vi "CH0_write_byte_data_and_sign_into_mem_no_g_Rev02x.vi"(0 "MB data":u8, 1 "UB data":u8, 2 "Address of the sign":string, 3 "USB Interface Name":refnum<visa-resource-name>="COM3", 4 "HB data":u8, 5 "LB data":u8, 6 "MB address":string, 7 "HB address":string, 8 "Sign Value":dbl, 9 "WRITE DATA":bool, 10 "Input buffer size":u32=16384, 11 "LB address":string, 12 "UB address":string, 13 "error in (no error)":errorcluster) -> (14 "MB data string":string, 15 "UB data string":string, 17 "error out":errorcluster, 18 "HB data string":string, 19 "LB data string":string)   [LabVIEW 2012]
panel:
  out "T command Bytes sent 5":dbl
  out "T command Bytes sent 4":dbl
  out "T command Bytes sent 3":dbl
  out "T command Bytes sent 2":dbl
  out "T command Bytes sent":dbl
  out "First 'T' Number of bytes written":dbl
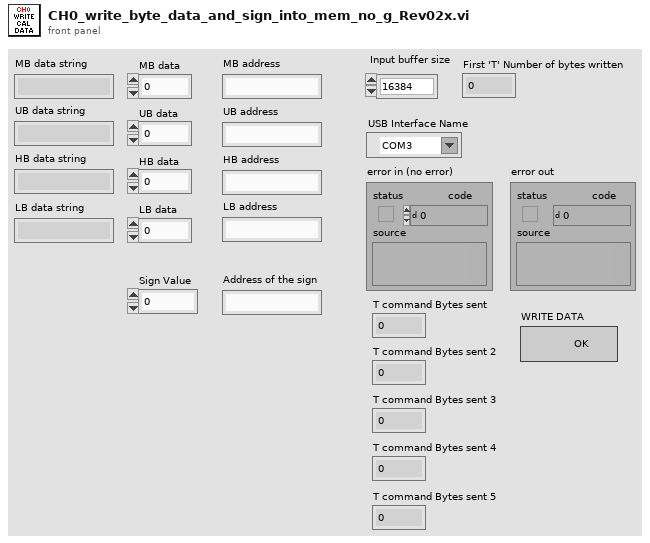
[diagram p1: front panel]
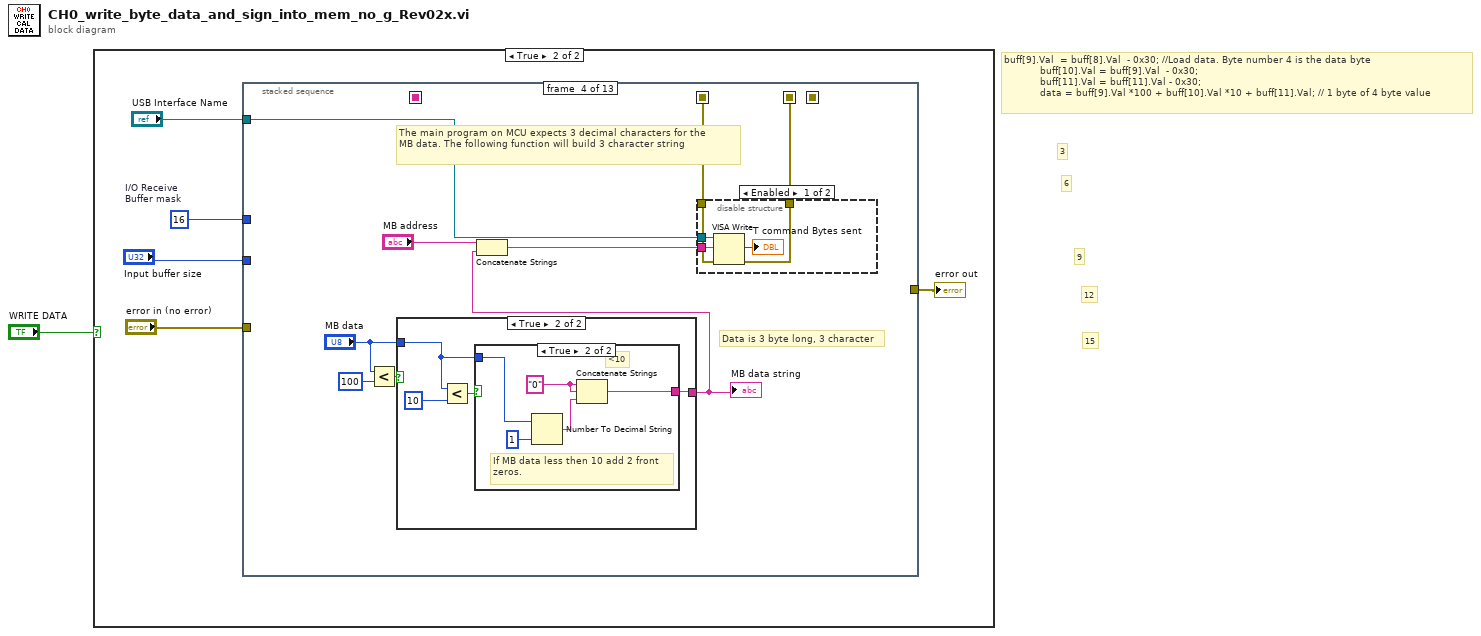
[diagram p0: block diagram]
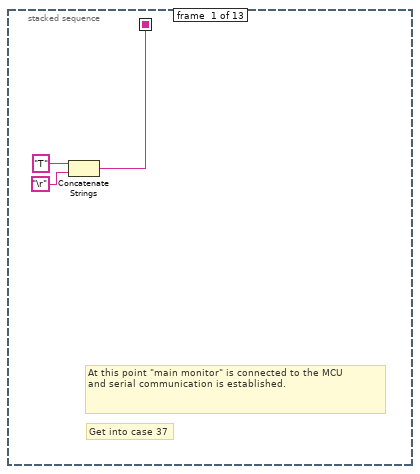
[diagram p3: hidden frame]
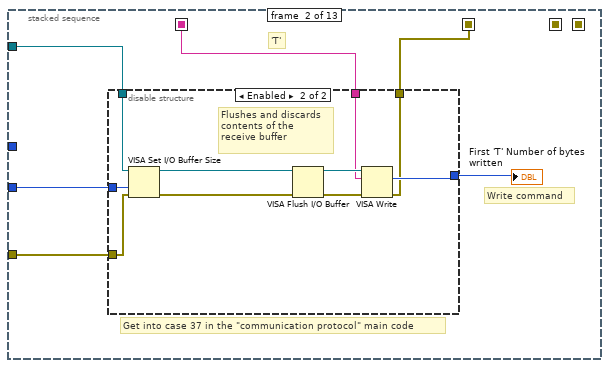
[diagram p4: hidden frame]
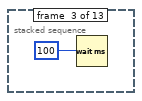
[diagram p6: hidden frame]
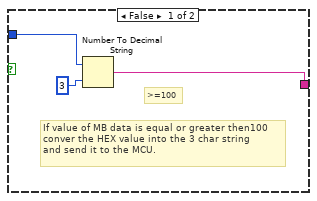
[diagram p7: hidden frame]
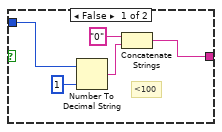
[diagram p8: hidden frame]
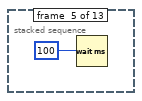
[diagram p10: hidden frame]
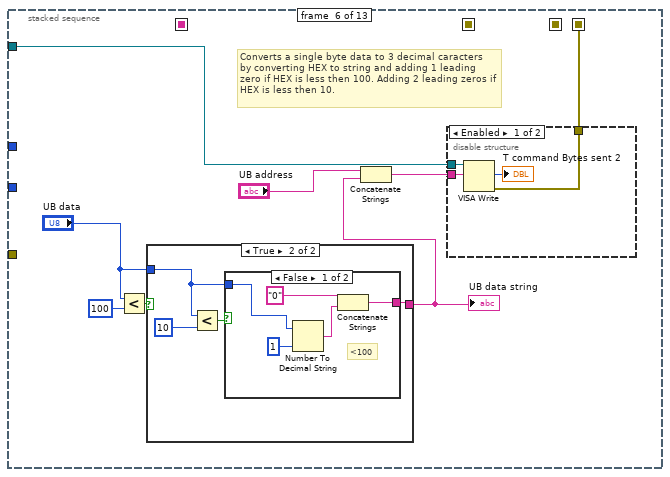
[diagram p11: hidden frame]
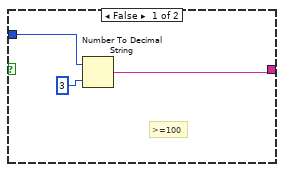
[diagram p12: hidden frame]
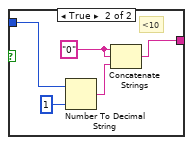
[diagram p13: hidden frame]
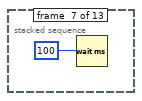
[diagram p15: hidden frame]
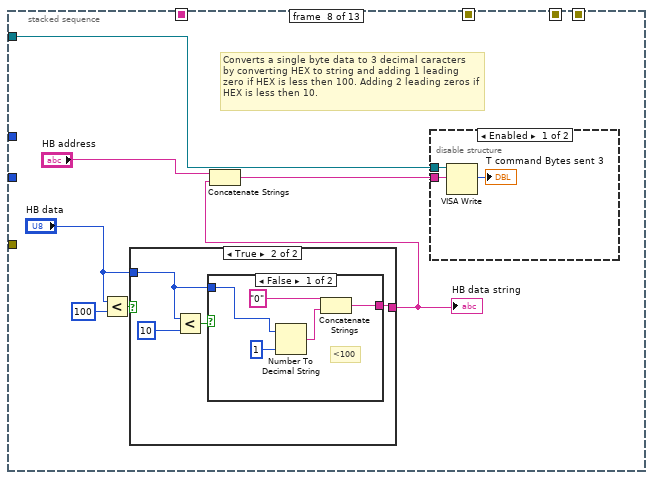
[diagram p16: hidden frame]
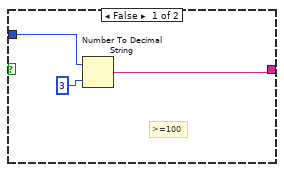
[diagram p17: hidden frame]
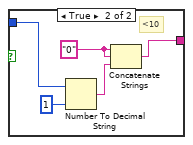
[diagram p18: hidden frame]
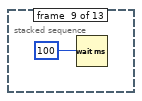
[diagram p20: hidden frame]
diagram:
  # "15"
  # "3"
  # "12"
  # "9"
  # "6"
  # "buff[9].Val  = buff[8].Val  - 0x30; //Load data. Byte number 4 is the data byte           \n            buff[10].Val = buff[9].Val  - 0x30;           \n            buff[11].Val = buff[11].Val - 0x30;               \n            data = buff[9].Val *100 + buff[10].Val *10 + buff[11].Val; // 1 byte of 4 byte value"
  n1 = case shown="True" "WRITE DATA" {
    frame False {
    }
    frame True {
      w4 = u16 16  # I/O Receive Buffer mask
      n2 = stacked-sequence {
        seq-local: [w7 _ _ _ _ _ _ _ _ _ _ _ _] -> [_ w12 _ _ _ _ _ _ _ _ _ _ _]
        seq-local: [_ w11 _ _ _ _ _ _ _ _ _ _ _] -> [_ _ _ w29 _ _ _ _ _ _ _ _ _]
        seq-local: [_ _ _ w28 _ _ _ _ _ _ _ _ _] -> [_ _ _ _ _ _ _ _ _ _ _ _ _]
        seq-local: [_ _ _ _ _ w60 _ _ _ _ _ _ _] -> [_ _ _ _ _ _ _ _ _ _ _ _ _]
        tunnel: "USB Interface Name" -> [_ w15 _ w34 _ w61 _ w90 _ w119 _ w153 w159]
        tunnel: "error in (no error)" -> [_ w14 _ _ _ _ _ _ _ _ _ _ _]
        tunnel: "Input buffer size" -> [_ w13 _ _ _ _ _ _ _ _ _ _ _]
        tunnel: w4 -> [_ _ _ _ _ _ _ _ _ _ _ _ _]
        tunnel: [_ _ _ _ _ _ _ _ _ w117 _ _ _] -> w3
        frame #0 {
          # "At this point \"main monitor\" is connected to the MCU\nand serial communication is established."
          # "Get into case 37"
          n3 = Concatenate Strings("T", "\r") -> (w7:string)
        }
        frame #1 {
          # "'T'"
          # "Get into case 37 in the \"communication protocol\" main code"
          # "Write command"
          n4 = disable-structure shown="Enabled" {
            disable-tunnel: w13 -> [_ w21]
            disable-tunnel: w12 -> [_ w20]
            disable-tunnel: w15 -> [_ w19]
            disable-tunnel: w14 -> [_ w18]
            disable-tunnel: [_ w17] -> w10
            disable-tunnel: [_ w16] -> w11
            frame Disabled {
            }
            frame Enabled {
              # "Flushes and discards \ncontents of the \nreceive buffer"
              n5 = VISA Set I/O Buffer Size(VISA resource name=w19, size (4096)=w21, error in (no error)=w18) -> (VISA resource name out=w23:refnum<visa-resource-name>, error out=w22:errorcluster)  [unwired: 1 in]
              n6 = VISA Flush I/O Buffer(VISA resource name=w23, error in (no error)=w22) -> (VISA resource name out=w25:refnum<visa-resource-name>, error out=w24:errorcluster)  [unwired: 1 in]
              n7 = VISA Write(VISA resource name=w25, write buffer=w20, error in (no error)=w24) -> (return count=w17:u32, error out=w16:errorcluster)  [unwired: 1 out]
            }
          }
          "First 'T' Number of bytes written" <- w10
        }
        frame #2 {
          n8 = Wait (ms)(milliseconds to wait=100) -> ()  [unwired: 1 out]
        }
        frame #3 {
          # "Data is 3 byte long, 3 character"
          # "The main program on MCU expects 3 decimal characters for the \nMB data. The following function will build 3 character string"
          n9 = Less?(x="MB data", y=100) -> (x < y?=w33:bool)
          n10 = case shown="True" w33 {
            tunnel: [w38 w39] -> w30
            tunnel: "MB data" -> [w36 w40]
            frame False {
              # "If value of MB data is equal or greater then100\nconver the HEX value into the 3 char string \nand send it to the MCU."
              # ">=100"
              n11 = Number To Decimal String(number=w36, width (-)=3) -> (decimal integer string=w38:string)
            }
            frame True {
              n12 = Less?(x=w40, y=10) -> (x < y?=w42:bool)
              n13 = case shown="True" w42 {
                tunnel: w40 -> [w45 w48]
                tunnel: [w44 w49] -> w39
                frame False {
                  # "<100"
                  n14 = Number To Decimal String(number=w45, width (-)=1) -> (decimal integer string=w46:string)
                  n15 = Concatenate Strings("0", w46) -> (w44:string)
                }
                frame True {
                  w50 = "0"
                  # "If MB data less then 10 add 2 front\nzeros."
                  # "<10"
                  n16 = Number To Decimal String(number=w48, width (-)=1) -> (decimal integer string=w51:string)
                  n17 = Concatenate Strings(w50, w50, w51) -> (w49:string)
                }
              }
            }
          }
          "MB data string" <- w30
          n18 = Concatenate Strings("MB address", w30) -> (w35:string)
          n19 = disable-structure shown="Enabled" {
            disable-tunnel: w35 -> [w56 _]
            disable-tunnel: w34 -> [w55 _]
            disable-tunnel: w29 -> [w54 _]
            disable-tunnel: [w53 _] -> w28
            frame Enabled {
              n20 = VISA Write(VISA resource name=w55, write buffer=w56, error in (no error)=w54) -> (return count=→"T command Bytes sent":u32, error out=w53:errorcluster)  [unwired: 1 out]
            }
            frame Disabled {
            }
          }
        }
        frame #4 {
          n21 = Wait (ms)(milliseconds to wait=100) -> ()  [unwired: 1 out]
        }
        frame #5 {
          # "Converts a single byte data to 3 decimal caracters\nby converting HEX to string and adding 1 leading zero if HEX is less then 100. Adding 2 leading zeros if HEX is less then 10."
          n22 = Less?(x="UB data", y=100) -> (x < y?=w65:bool)
          n23 = case shown="True" w65 {
            tunnel: [w69 w70] -> w62
            tunnel: "UB data" -> [w67 w71]
            frame False {
              # ">=100"
              n24 = Number To Decimal String(number=w67, width (-)=3) -> (decimal integer string=w69:string)
            }
            frame True {
              n25 = Less?(x=w71, y=10) -> (x < y?=w73:bool)
              n26 = case shown="False" w73 {
                tunnel: w71 -> [w75 w79]
                tunnel: [w74 w80] -> w70
                frame False {
                  # "<100"
                  n27 = Number To Decimal String(number=w75, width (-)=1) -> (decimal integer string=w76:string)
                  n28 = Concatenate Strings("0", w76) -> (w74:string)
                }
                frame True {
                  w81 = "0"
                  # "<10"
                  n29 = Number To Decimal String(number=w79, width (-)=1) -> (decimal integer string=w82:string)
                  n30 = Concatenate Strings(w81, w81, w82) -> (w80:string)
                }
              }
            }
          }
          "UB data string" <- w62
          n31 = Concatenate Strings("UB address", w62) -> (w66:string)
          n32 = disable-structure shown="Enabled" {
            disable-tunnel: w66 -> [w86 _]
            disable-tunnel: w61 -> [w85 _]
            disable-tunnel: [w84 _] -> w60
            frame Enabled {
              n33 = VISA Write(VISA resource name=w85, write buffer=w86) -> (return count=→"T command Bytes sent 2":u32, error out=w84:errorcluster)  [unwired: 1 in, 1 out]
            }
            frame Disabled {
            }
          }
        }
        frame #6 {
          n34 = Wait (ms)(milliseconds to wait=100) -> ()  [unwired: 1 out]
        }
        frame #7 {
          # "Converts a single byte data to 3 decimal caracters\nby converting HEX to string and adding 1 leading zero if HEX is less then 100. Adding 2 leading zeros if HEX is less then 10."
          n35 = Less?(x="HB data", y=100) -> (x < y?=w94:bool)
          n36 = case shown="True" w94 {
            tunnel: [w98 w99] -> w91
            tunnel: "HB data" -> [w96 w100]
            frame False {
              # ">=100"
              n37 = Number To Decimal String(number=w96, width (-)=3) -> (decimal integer string=w98:string)
            }
            frame True {
              n38 = Less?(x=w100, y=10) -> (x < y?=w102:bool)
              n39 = case shown="False" w102 {
                tunnel: w100 -> [w104 w108]
                tunnel: [w103 w109] -> w99
                frame False {
                  # "<100"
                  n40 = Number To Decimal String(number=w104, width (-)=1) -> (decimal integer string=w105:string)
                  n41 = Concatenate Strings("0", w105) -> (w103:string)
                }
                frame True {
                  w110 = "0"
                  # "<10"
                  n42 = Number To Decimal String(number=w108, width (-)=1) -> (decimal integer string=w111:string)
                  n43 = Concatenate Strings(w110, w110, w111) -> (w109:string)
                }
              }
            }
          }
          "HB data string" <- w91
          n44 = Concatenate Strings("HB address", w91) -> (w95:string)
          n45 = disable-structure shown="Enabled" {
            disable-tunnel: w95 -> [w114 _]
            disable-tunnel: w90 -> [w113 _]
            frame Enabled {
              n46 = VISA Write(VISA resource name=w113, write buffer=w114) -> (return count=→"T command Bytes sent 3":u32)  [unwired: 1 in, 2 out]
            }
            frame Disabled {
            }
          }
        }
        frame #8 {
          n47 = Wait (ms)(milliseconds to wait=100) -> ()  [unwired: 1 out]
        }
        frame #9 {
          # "The main program on MCU expects 3 decimal characters for the \nMB data. The following function will build 3 character string"
          n48 = Less?(x="LB data", y=100) -> (x < y?=w123:bool)
          n49 = case shown="True" w123 {
            tunnel: [w127 w128] -> w120
            tunnel: "LB data" -> [w125 w129]
            frame False {
              # ">=100"
              n50 = Number To Decimal String(number=w125, width (-)=3) -> (decimal integer string=w127:string)
            }
            frame True {
              n51 = Less?(x=w129, y=10) -> (x < y?=w131:bool)
              n52 = case shown="True" w131 {
                tunnel: w129 -> [w133 w137]
                tunnel: [w132 w138] -> w128
                frame False {
                  # "<100"
                  n53 = Number To Decimal String(number=w133, width (-)=1) -> (decimal integer string=w134:string)
                  n54 = Concatenate Strings("0", w134) -> (w132:string)
                }
                frame True {
                  w139 = "0"
                  # "<10"
                  n55 = Number To Decimal String(number=w137, width (-)=1) -> (decimal integer string=w140:string)
                  n56 = Concatenate Strings(w139, w139, w140) -> (w138:string)
                }
              }
            }
          }
          "LB data string" <- w120
          n57 = Concatenate Strings("LB address", w120) -> (w124:string)
          n58 = disable-structure shown="Enabled" {
            disable-tunnel: w124 -> [w144 _]
            disable-tunnel: w119 -> [w143 _]
            disable-tunnel: [w142 _] -> w117
            frame Enabled {
              n59 = VISA Write(VISA resource name=w143, write buffer=w144) -> (return count=→"T command Bytes sent 4":u32, error out=w142:errorcluster)  [unwired: 1 in, 1 out]
            }
            frame Disabled {
            }
          }
        }
        frame #10 {
          n60 = Wait (ms)(milliseconds to wait=100) -> ()  [unwired: 1 out]
        }
        frame #11 {
          w150 = "0"
          # "001 or 000"
          # "<10"
          n61 = Number To Decimal String(number="Sign Value", width (-)=1) -> (decimal integer string=w151:string)
          n62 = Concatenate Strings(w150, w150, w151) -> (w148:string)
          n63 = Concatenate Strings("Address of the sign", w148) -> (w154:string)
          n64 = disable-structure shown="Enabled" {
            disable-tunnel: w154 -> [w157 _]
            disable-tunnel: w153 -> [w156 _]
            disable-tunnel: [w155 _] -> _
            frame Enabled {
              n65 = VISA Write(VISA resource name=w156, write buffer=w157) -> (return count=→"T command Bytes sent 5":u32, error out=w155:errorcluster)  [unwired: 1 in, 1 out]
            }
            frame Disabled {
            }
          }
        }
        frame #12 {
          # "Reset instrument"
          n66 = call "g_send.vi"("Input buffer size"=16384, "USB Interface Name"=w159) -> ()  [unwired: 9 in, 1 out]
        }
      }
      "error out" <- w3
    }
  }
